vi "Begin.vi"(8 "error in (no error)":errorcluster, 10 "Config In":variant, 11 "Falcon500 in":refnum<class "Falcon500.lvclass">) -> (0 "error out":errorcluster, 3 "Falcon500 out":refnum<class "Falcon500.lvclass">)   [LabVIEW 2019, in "Drive.lvlib" / "Falcon500.lvclass"]
uses:
  Falcon500.lvclass
  C:/Users/Public/Documents/2020InfinteRecharge/src robot/Classes/Drive/Tank Drive/Tank Drive.lvclass
  Controls/PIDF.ctl
  941a1825-4eaa-4cb3-98e1-62e177f30608.vi
  228b2b1e-43de-4b58-a042-7794822295de.vi
  <vilib>/Utility/error.llb/Trim Whitespace.vi
  <vilib>/Utility/error.llb/Error Cluster From Error Code.vi
  CTRE Drive.lvclass
  Tank Drive.lvclass
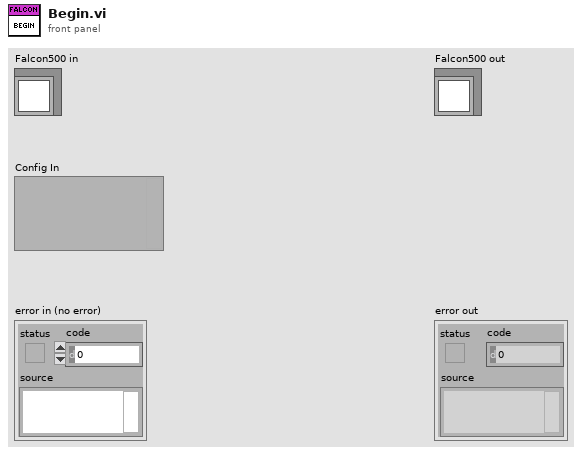
[diagram p1: front panel]
types:
  T1 = typedef "Drive.lvlib/Tank Drive.lvclass/PIDF.ctl" = cluster{"P":dbl, "I":dbl, "D":dbl, "F":dbl}
  T2 = typedef "Drive.lvlib/Tank Drive.lvclass/Motor Controller IDs.ctl" = cluster{"Left Lead":u8, "Right Lead":u8, "Left Followers":u8[], "Right Followers":u8[]}
  T3 = typedef "Drive.lvlib/Tank Drive.lvclass/Motor Controller Names.ctl" = cluster{"Left Lead":string, "Right Lead":string, "Left Followers":string[], "Right Followers":string[]}
  T4 = typedef "Drive.lvlib/Tank Drive.lvclass/Constants.ctl" = cluster{"Drive Velocity Low Gear":T5, "Drive Velocity High Gear":T5, "Drive Motion Magic Primary Low Gear":T5, "Drive Motion Magic Primary High Gear":T5, "Drive Motion Magic Secondary Low Gear":T5, "Drive Motion Magic Secondary High Gear":T5, "Drive Sensors":T6, "Motion Magic Constants":T7, "Supply Current Limit Configuration":T8}
  T5 = typedef "CTRE_Phoenix_MotorControl_SlotStructure.ctl" = cluster{"P":dbl, "I":dbl, "D":dbl, "F":dbl, "integralZone":dbl, "allowableClosedLoopError":i32, "maxIntegralAccumulator":dbl, "closedLoopPeakOutput":dbl, "closedLoopPeriod":i32}
  T6 = typedef "DriveOld.lvlib/Drive.lvclass/Drive Sensor Data.ctl" = cluster{"Drive Right Invert":bool, "Drive Right Sensor Phase":bool, "Drive Left Invert":bool, "Drive Left Sensor Phase":bool}
  T7 = typedef "DriveOld.lvlib/Drive.lvclass/Motion Magic Constants.ctl" = cluster{"Low Gear Max Velocity":u32, "High Gear Max Velocity":u32, "Motion Magic Low Gear Max Velocity":u32, "Motion Magic Low Gear Max Acceleration":u32, "Motion Magic High Gear Max Velocity":u32, "Motion Magic High Gear Max Acceleration":u32}
  T8 = typedef "CTRE_Phoenix_MotorControl_SupplyCurrentLimitConfiguration.ctl" = cluster{"Enable?":bool, "Current Limit":dbl, "Threshold Current":dbl, "Threshold Time":dbl}
  T9 = typedef "WPI_MotorControlDeviceRef.ctl" = cluster{"DeviceStatus":errorcluster, "Type":T10, "PWM":cluster{"PWM Channel":T11, "DeadBand":T12}, "CAN":cluster{"Device Number":u8, "SetOutput VI Ref":variant, "GetOutput VI Ref":variant, "Enable VI Ref":variant, "Disable VI Ref":variant, "Data":variant}, "Invert":bool, "DIO PWM":cluster{"PWM \"Enable\" Channel":T11, "DIOChannel":T13, "PWM Rate":dbl}}
  T10 = typedef "WPI_MotorControlType.ctl" = enum16{"PWM", "CAN", "DIO PWM"}
  T11 = typedef "FPGA_DIOPWMChannel.ctl" = enum8{"PWM 0", "PWM 1", "PWM 2", "PWM 3", "PWM 4", "PWM 5", "PWM 6", "PWM 7", "PWM 8", "PWM 9", "PWM MXP 0", "PWM MXP 1", "PWM MXP 2", "PWM MXP 3", "PWM MXP 4", "PWM MXP 5", "PWM MXP 6", "PWM MXP 7", "PWM MXP 8", "PWM MXP 9", "Invalid"}
  T12 = typedef "WPI_PWMDeadband.ctl" = cluster{"Name":string, "maxPositivePwm":i32, "minPositivePwm":i32, "centerPwm":i32, "maxNegativePwm":i32, "minNegativePwm":i32, "angularRange":u16}
  T13 = typedef "FPGA_DIOChannel.ctl" = enum8{"DIO 0", "DIO 1", "DIO 2", "DIO 3", "DIO 4", "DIO 5", "DIO 6", "DIO 7", "DIO 8", "DIO 9", "DIO MXP 0", "DIO MXP 1", "DIO MXP 2", "DIO MXP 3", "DIO MXP 4", "DIO MXP 5", "DIO MXP 6", "DIO MXP 7", "DIO MXP 8", "DIO MXP 9", "DIO MXP 10", "DIO MXP 11", "DIO MXP 12", "DIO MXP 13", "DIO MXP 14", "DIO MXP 15", "SPI Port CS1", "SPI Port CS2", "SPI Port CS3", "SPI Port MISO", "SPI Port MOSI", "Invalid"}
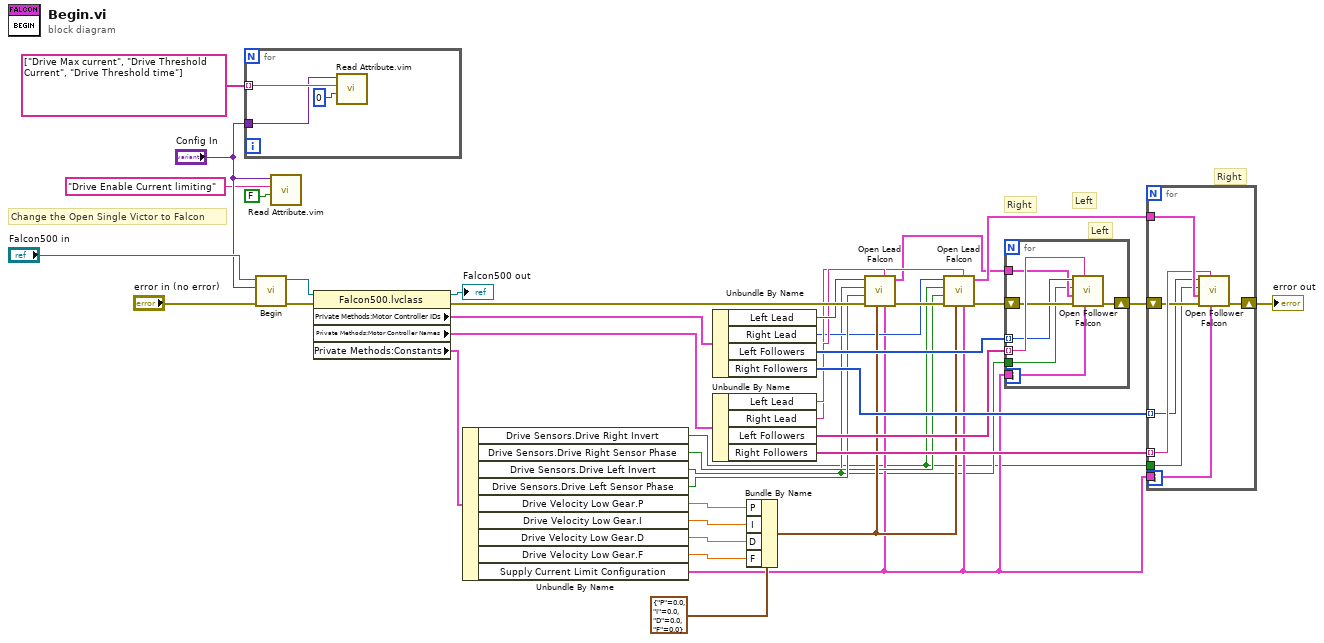
[diagram p0: block diagram]
diagram:
  # "Right"
  # "Left"
  # "Right"
  # "Left"
  # "Change the Open Single Victor to Falcon"
  n1 = for {
    tunnel: string[] ["Drive Max current", "Drive Threshold Current", "Drive Threshold time"] -> [w41] mode=indexing
    tunnel: "Config In" -> [w39]
    n2 = call "Read Attribute.vim"("default value (data type)"=u8 0, "name"=w41, "variant in"=w39) -> ()  [unwired: 5 in, 4 out]
  }
  n3 = call-parent "Begin.vi"("error in (no error)"="error in (no error)", "Config In"="Config In", "Tank Drive in"="Falcon500 in") -> ("error out"=w29:errorcluster, "Tank Drive out"=w26:refnum<class "Falcon500.lvclass">)  [unwired: 7 in]
  n4 = call "Read Attribute.vim"("default value (data type)"=FALSE, "name"="Drive Enable Current limiting", "variant in"="Config In") -> ()  [unwired: 5 in, 4 out]
  n5 = property class="Falcon500.lvclass"(reference=w26, error in=w29) -> (reference out=→"Falcon500 out":refnum<class "Falcon500.lvclass">, error out=w16:errorcluster, "Private Methods:Motor Controller IDs"=w37:T2, "Private Methods:Motor Controller Names"=w36:T3, "Private Methods:Constants"=w21:T4)
  n6 = Unbundle By Name(w21) -> ("Drive Sensors.Drive Right Invert"=w1:bool, "Drive Sensors.Drive Right Sensor Phase"=w7:bool, "Drive Sensors.Drive Left Invert"=w2:bool, "Drive Sensors.Drive Left Sensor Phase"=w15:bool, "Drive Velocity Low Gear.P"=w20:dbl, "Drive Velocity Low Gear.I"=w19:dbl, "Drive Velocity Low Gear.D"=w18:dbl, "Drive Velocity Low Gear.F"=w17:dbl, "Supply Current Limit Configuration"=w4:T8)
  n7 = Unbundle By Name(w37) -> ("Left Lead"=w14:u8, "Right Lead"=w6:u8, "Left Followers"=w35:u8[], "Right Followers"=w34:u8[])
  n8 = Unbundle By Name(w36) -> ("Left Lead"=w12:string, "Right Lead"=w8:string, "Left Followers"=w33:string[], "Right Followers"=w32:string[])
  n9 = Bundle By Name(cluster=T1 {"P"=0.0, "I"=0.0, "D"=0.0, "F"=0.0} ("PIDF Constants"), "P"=w20, "I"=w19, "D"=w18, "F"=w17) -> (w9:T1)
  n10 = call "Open Lead Falcon.vi"("can id"=w14, "Drive Invert"=w2, "Drive Sensor Phase"=w15, "error in (no error)"=w16, "PIDF Constants"=w9, "refnum name"=w12, "Supply Current Limit Configuration"=w4) -> ("PhoenixMotorControlDevRef"=w3:T9, "error out"=w11:errorcluster)  [unwired: 2 in]
  n11 = call "Open Lead Falcon.vi"("can id"=w6, "Drive Invert"=w1, "Drive Sensor Phase"=w7, "error in (no error)"=w11, "PIDF Constants"=w9, "refnum name"=w8, "Supply Current Limit Configuration"=w4) -> ("PhoenixMotorControlDevRef"=w5:T9, "error out"=w10:errorcluster)  [unwired: 2 in]
  n12 = for {
    tunnel: w35 -> [w45] mode=indexing
    tunnel: w33 -> [w48] mode=indexing
    shift-right: [w46] -> w28
    shift-left: w10 -> [w47]
    tunnel: w4 -> [w44]
    tunnel: w3 -> [w43]
    tunnel: w2 -> [w42]
    n13 = call "Open Follower Falcon.vi"("Supply Current Limit Configuration"=w44, "refnum name"=w48, "error in (no error)"=w47, "Master Controller to Follow"=w43, "Invert?"=w42, "Device Number"=w45) -> ("error out"=w46:errorcluster)  [unwired: 5 in]
  }
  n14 = for {
    tunnel: w34 -> [w50] mode=indexing
    tunnel: w32 -> [w54] mode=indexing
    shift-right: [w52] -> w27
    shift-left: w28 -> [w53]
    tunnel: w5 -> [w55]
    tunnel: w4 -> [w51]
    tunnel: w1 -> [w49]
    n15 = call "Open Follower Falcon.vi"("Supply Current Limit Configuration"=w51, "refnum name"=w54, "error in (no error)"=w53, "Master Controller to Follow"=w55, "Invert?"=w49, "Device Number"=w50) -> ("error out"=w52:errorcluster)  [unwired: 5 in]
  }
  "error out" <- w27
